vi "ChannelListGenerator.vi"(10 "Card Type":enum16{"7036", "7054"}(ring), 11 "Channels":i32[](array[numeric])) -> (2 "Channel List":T1(array[cluster]))   [LabVIEW 2019]
uses:
  globals/QC_MeasurementSetup.vi
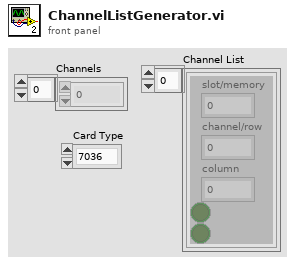
[diagram p1: front panel]
types:
  T1 = cluster{"slot/memory":i16, "channel/row":i16, "column":i16, bool, bool}[]
  T2 = cluster{"slot/memory":i16, "channel/row":i16, "column":i16, bool, bool}
  T3 = cluster{"User":string, " Institute":string, " Test Time":string, " Test Date":string, "Instruments":string, "Sensor Serials":string[], "IV Test?":bool, "CV Test? ":bool, "LCS Test? ":bool, "No. of Ch.":u16, " Current Sensor":string, " Current Test":string, "Arduino DP Map":string[], "Sensor DB IDs":string[], "Sensor Types":string[], "Data directory":string, "7036 Channel Map":string[], "7054 1 Map":string[], "7054 2 Map ":string[], "7054 3 Map ":string[], "Data Paths":string[][], "IV":bool[], "CV":bool[], "Stability":bool[]}
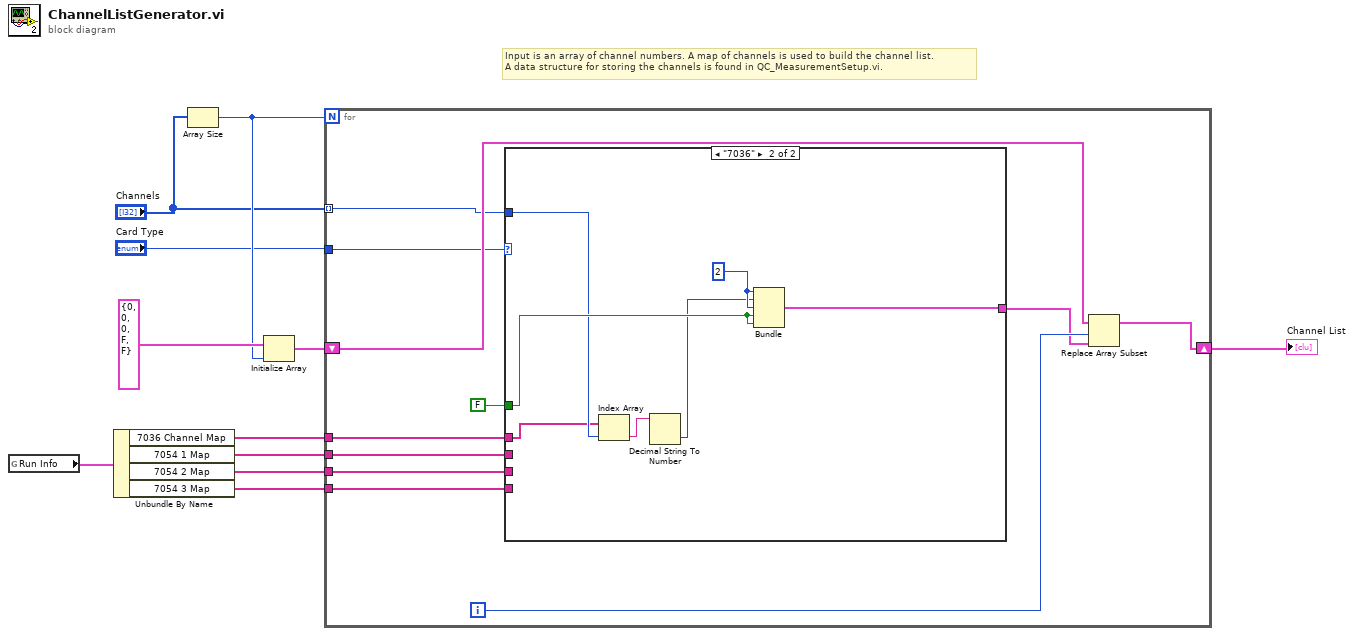
[diagram p0: block diagram]
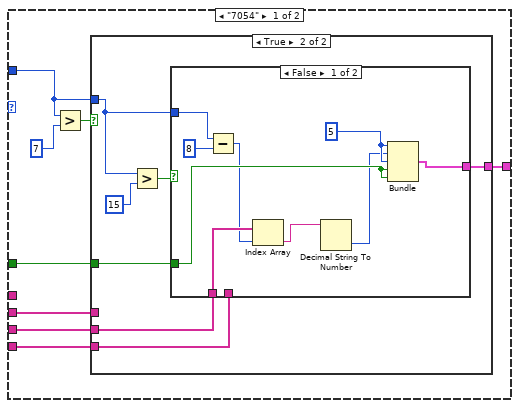
[diagram p2: hidden frame]
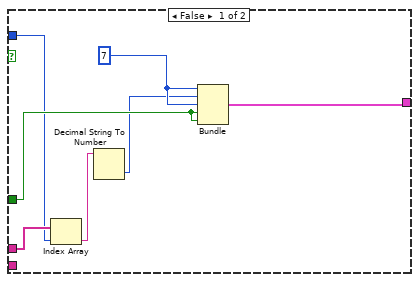
[diagram p3: hidden frame]
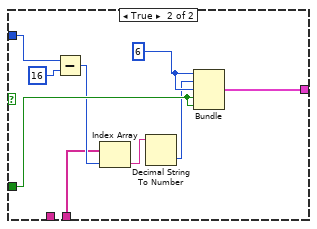
[diagram p4: hidden frame]
diagram:
  # "Input is an array of channel numbers. A map of channels is used to build the channel list. \nA data structure for storing the channels is found in QC_MeasurementSetup.vi."
  n1 = global read "QC_MeasurementSetup.vi" "Run Info"() -> (w6:T3)
  n2 = Unbundle By Name(w6) -> ("7036 Channel Map"=w5:string[], "7054 1 Map"=w4:string[], "7054 2 Map"=w3:string[], "7054 3 Map"=w2:string[])
  n3 = Array Size(array="Channels") -> (size(s)=w9:i32)
  n4 = Initialize Array(T2 {"slot/memory"=0, "channel/row"=0, "column"=0, FALSE, FALSE} ("channel definition"), w9) -> (w10:T1)
  n5 = for {
    N: w9 -> [_]
    shift-right: [w18] -> w7
    shift-left: w10 -> [w19]
    tunnel: "Card Type" -> [w17]
    tunnel: w5 -> [w16]
    tunnel: w4 -> [w14]
    tunnel: w3 -> [w13]
    tunnel: w2 -> [w12]
    tunnel: "Channels" -> [w15] mode=indexing
    i -> [w21]
    n6 = case shown="\"7036\"" w17 {
      tunnel: FALSE -> [w28 w67]
      tunnel: [w27 w69] -> w20
      tunnel: w16 -> [_ w64]
      tunnel: w15 -> [w26 w65]
      tunnel: w14 -> [w25 _]
      tunnel: w13 -> [w24 _]
      tunnel: w12 -> [w23 _]
      frame "7054" {
        n7 = Greater?(x=w26, y=7) -> (0:w30:bool)
        n8 = case shown="True" w30 {
          tunnel: w28 -> [w36 w42]
          tunnel: w26 -> [w32 w38]
          tunnel: [w35 w41] -> w27
          tunnel: w25 -> [w33 _]
          tunnel: w24 -> [_ w40]
          tunnel: w23 -> [_ w39]
          frame False {
            w37 = 7
            n9 = Index Array(array=w33, index=w32) -> (element=w31:string)
            n10 = Decimal String To Number(string=w31) -> (number=w34:i32)  [unwired: 2 in, 1 out]
            n11 = Bundle(w37, w34, w37, w36, w36) -> (w35:cluster{i32, i32, i32, bool, bool})  [unwired: 1 in]
          }
          frame True {
            n12 = Greater?(x=w38, y=15) -> (0:w43:bool)
            n13 = case shown="False" w43 {
              tunnel: w42 -> [w52 w61]
              tunnel: [w51 w60] -> w41
              tunnel: w40 -> [w49 _]
              tunnel: w39 -> [_ w55]
              tunnel: w38 -> [w48 w56]
              frame False {
                w53 = 5
                n14 = Subtract(x=w48, y=8) -> (x-y=w47:i32)
                n15 = Index Array(array=w49, index=w47) -> (element=w45:string)
                n16 = Decimal String To Number(string=w45) -> (number=w50:i32)  [unwired: 2 in, 1 out]
                n17 = Bundle(w53, w50, w53, w52, w52) -> (w51:cluster{i32, i32, i32, bool, bool})  [unwired: 1 in]
              }
              frame True {
                w62 = 6
                n18 = Subtract(x=w56, y=16) -> (x-y=w58:i32)
                n19 = Index Array(array=w55, index=w58) -> (element=w54:string)
                n20 = Decimal String To Number(string=w54) -> (number=w59:i32)  [unwired: 2 in, 1 out]
                n21 = Bundle(w62, w59, w62, w61, w61) -> (w60:cluster{i32, i32, i32, bool, bool})  [unwired: 1 in]
              }
            }
          }
        }
      }
      frame "7036" {
        w68 = 2
        n22 = Index Array(array=w64, index=w65) -> (element=w63:string)
        n23 = Decimal String To Number(string=w63) -> (number=w66:i32)  [unwired: 2 in, 1 out]
        n24 = Bundle(w68, w66, w68, w67, w67) -> (w69:cluster{i32, i32, i32, bool, bool})  [unwired: 1 in]
      }
    }
    n25 = Replace Array Subset(array=w19, new element=w20, index=w21) -> (w18:T1)
  }
  "Channel List" <- w7
